vi "DAQGEN_Trigger.vi"() -> ()   [LabVIEW 2016]
uses:
  <vilib>/rvi/Emulation/niFpgaGetClockAttributes.vi
  <vilib>/rvi/Emulation/niFpgaSctlEmulationGetInTimedLoop.vi
  <vilib>/rvi/Emulation/niFpgaEmulationReportErrorSimple.vi
  <vilib>/rvi/eio/common/nirviEmuTemplateMethod_errors.vi
  <vilib>/rvi/interface/RandomDataEmulation/niFpgaRandomDataHandleErrors.vi
  <vilib>/rvi/Emulation/niFpgaCriticalErrorInLSC.vi
  <vilib>/eio/EIONode/EIONode.xnode
  <vilib>/rvi/DataTransferAndStorage/Container/XNode/niFpgaContainer.xnode
  <vilib>/rvi/interface/RandomDataEmulation/nirviRandomDataFpgaReadWriteTemplate.vi
panel:
  in  "Sampling Rate (Hz)":i16=1000
  in  "# Samples":i16=10000
  in  "Wavegen!":bool
  in  "Stop DAQ":bool
  in  "Count(Ticks)":u32=500000
  out "Triggered?":bool
  in  "Pseudo Trigger":bool
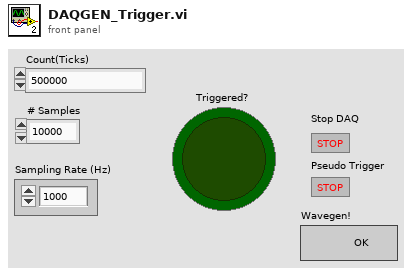
[diagram p1: front panel]
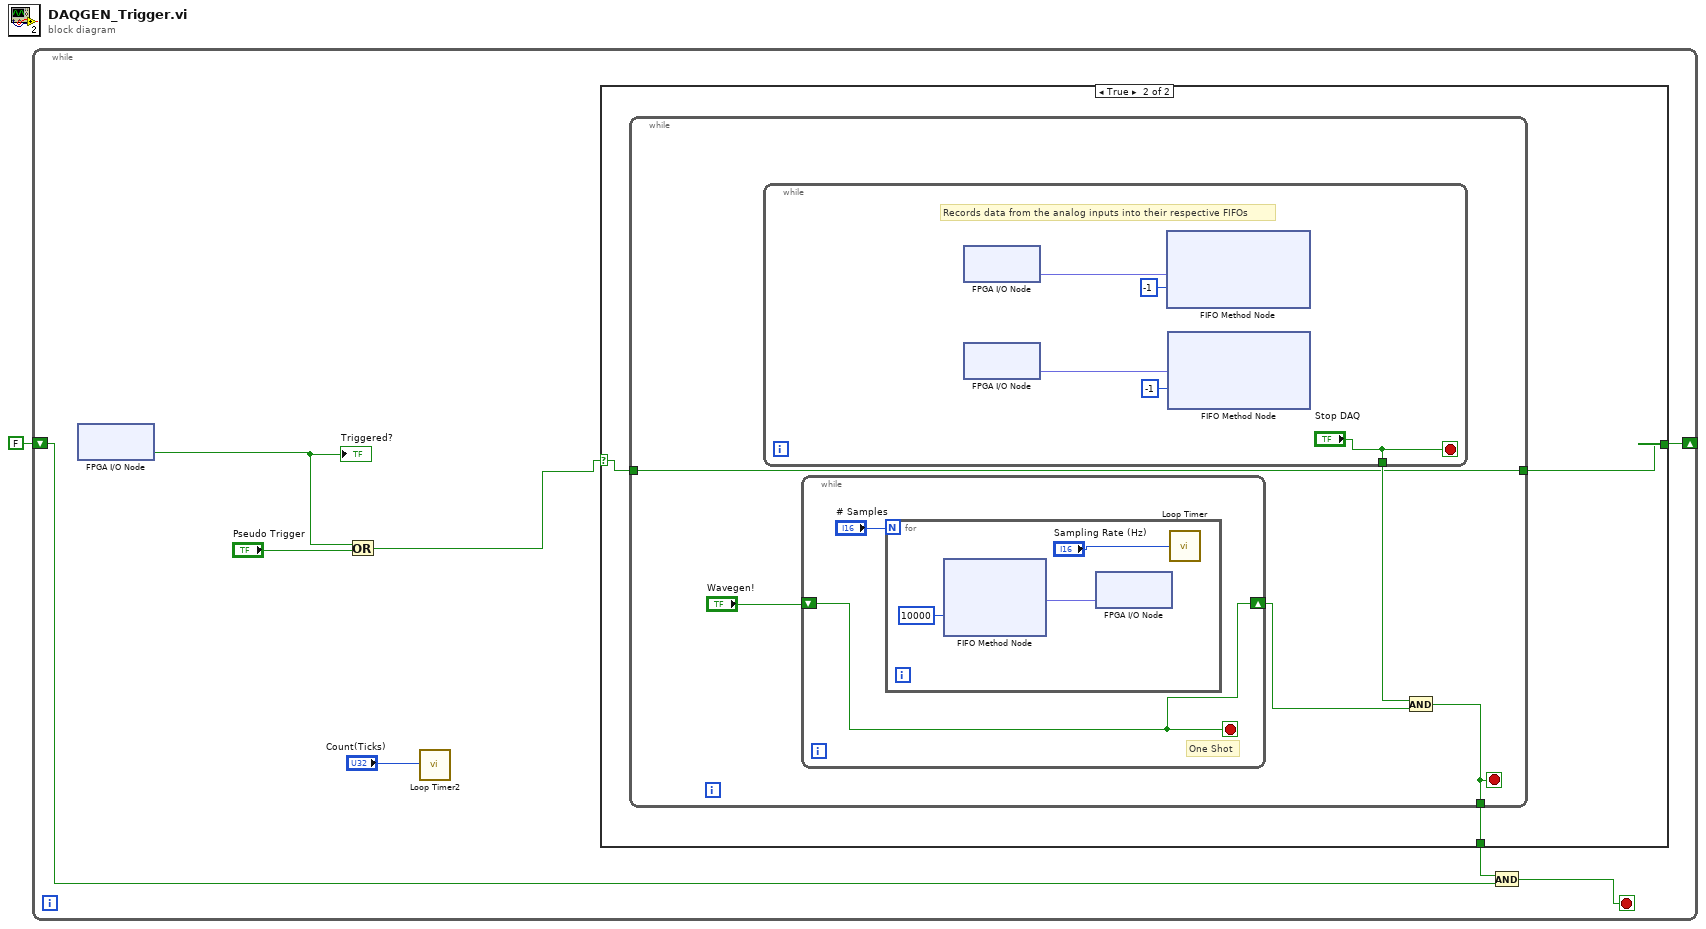
[diagram p0: block diagram]
diagram:
  n1 = while {
    shift-right: [w6] -> _
    shift-left: FALSE -> [w4]
    stop <- w3 stop-if-true
    n2 = xnode "FPGA I/O Node"() -> ("DIO3"=w8:bool)  [unwired: 1 in, 1 out]
    "Triggered?" <- w8
    n3 = Or(x=w8, y="Pseudo Trigger") -> (x .or. y?=w7:bool)
    n4 = call "Loop Timer2"("Count(Ticks)"="Count(Ticks)") -> ()  [unwired: 1 out]
    n5 = case shown="True" w7 {
      selector: w7 -> [w10 w11]
      tunnel: [w10 w12] -> w6
      tunnel: [w10 w13] -> w5
      frame False {
      }
      frame True {
        n6 = while {
          tunnel: [w15] -> w13
          tunnel: [w14] -> w12
          tunnel: w11 -> [w14]
          stop <- w15 stop-if-true
          n7 = while {
            tunnel: ["Stop DAQ"] -> w16
            stop <- "Stop DAQ" stop-if-true
            # "Records data from the analog inputs into their respective FIFOs"
            n8 = xnode "FPGA I/O Node"() -> ("AI0"=w23:fxp<+,16,3>)  [unwired: 1 in, 1 out]
            n9 = xnode "FPGA I/O Node"() -> ("AI7"=w22:fxp<+,16,3>)  [unwired: 1 in, 1 out]
            n10 = xnode ("FIFO Method Node")("Element"=w23, "Timeout"=-1) -> ()  [unwired: 1 in, 2 out]
            n11 = xnode ("FIFO Method Node")("Element"=w22, "Timeout"=-1) -> ()  [unwired: 1 in, 2 out]
          }
          n12 = while {
            shift-right: [w25] -> w17
            shift-left: "Wavegen!" -> [w25]
            stop <- w25 stop-if-true
            # "One Shot"
            n13 = for {
              N: "# Samples" -> [_]
              n14 = xnode ("FIFO Method Node")("Timeout"=10000) -> ("Element"=w27:fxp<+,16,3>)  [unwired: 1 in, 2 out]
              n15 = xnode "FPGA I/O Node"("AO0"=w27) -> ()  [unwired: 1 in, 1 out]
              n16 = call "Loop Timer"("Count(Ticks)"="Sampling Rate (Hz)") -> ()  [unwired: 1 out]
            }
          }
          n17 = And(x=w16, y=w17) -> (x .and. y?=w15:bool)
        }
      }
    }
    n18 = And(x=w5, y=w4) -> (x .and. y?=w3:bool)
  }
